vi "Sub_VI_Aleatorio-Sensores.vi"(10 "Altura da água":dbl, 11 "Havia erro?":bool) -> (2 "Altura final água":dbl, 3 "Boolean out":bool)   [LabVIEW 2019]
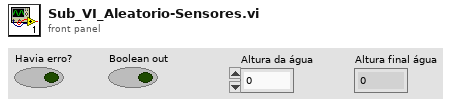
[diagram p1: front panel]
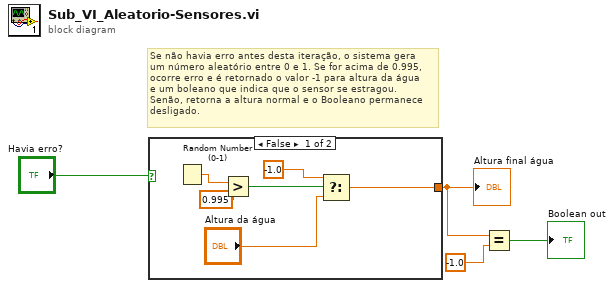
[diagram p0: block diagram]
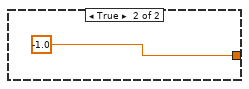
[diagram p2: hidden frame]
diagram:
  # "Se não havia erro antes desta iteração, o sistema gera\num número aleatório entre 0 e 1. Se for acima de 0.995,\nocorre erro e é retornado o valor -1 para altura da água\ne um boleano que indica que o sensor se estragou.\nSenão, retorna a altura normal e o Booleano permanece\ndesligado."
  n1 = case shown="False" "Havia erro?" {
    tunnel: [w6 -1.0] -> w3
    frame False {
      n2 = Random Number (0-1)() -> (number: 0 to 1=w9:dbl)
      n3 = Greater?(x=w9, y=0.995) -> (0:w8:bool)
      n4 = Select(t=-1.0, s=w8, f="Altura da água") -> (s? t:f=w6:dbl)
    }
    frame True {
    }
  }
  "Altura final água" <- w3
  n5 = Equal?(x=w3, y=-1.0) -> (x = y?=→"Boolean out":bool)
